vi "Get Time.vi"(8 "error in (no error)":errorcluster, 10 "Time Format (Absolute Time)":bool, 11 "VISA resource name":refnum<visa-resource-name>) -> (0 "error out":errorcluster, 1 "Current Time":string, 2 "Absolute Time":dbl format="%^#.8g", 3 "VISA resource name out":refnum<visa-resource-name>)   [LabVIEW 2020, in "Keithley 2450.lvlib"]
doc: "This gets the System Time in absolute or current time formats."
uses:
  Keithley 2450.lvlib
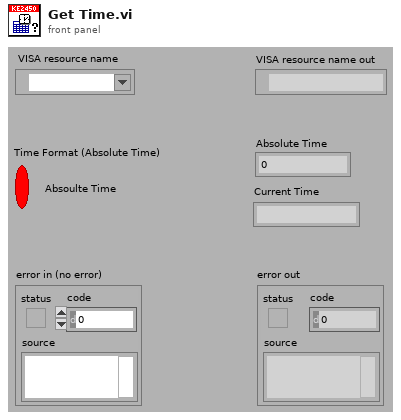
[diagram p1: front panel]
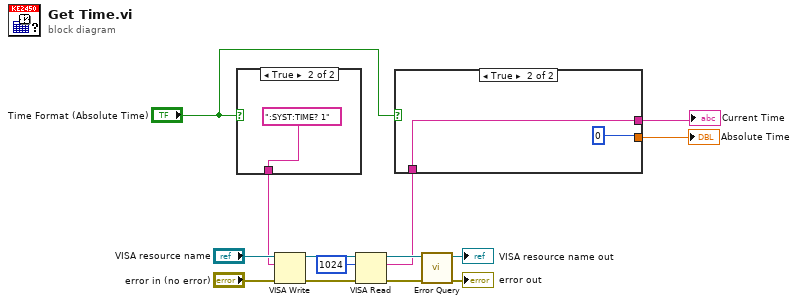
[diagram p0: block diagram]
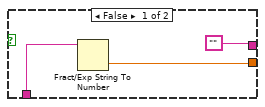
[diagram p2: hidden frame]
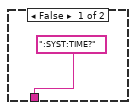
[diagram p3: hidden frame]
diagram:
  n1 = case shown="True" "Time Format (Absolute Time)" {
    tunnel: [":SYST:TIME?" ":SYST:TIME? 1"] -> w5
    frame False {
    }
    frame True {
    }
  }
  n2 = VISA Write(VISA resource name="VISA resource name", write buffer=w5, error in (no error)="error in (no error)") -> (VISA resource name out=w13:refnum<visa-resource-name>, error out=w14:errorcluster)  [unwired: 1 out]
  n3 = VISA Read(VISA resource name=w13, byte count=u32 1024, error in (no error)=w14) -> (VISA resource name out=w7:refnum<visa-resource-name>, read buffer=w4:string, error out=w6:errorcluster)  [unwired: 1 out]
  n4 = case shown="True" "Time Format (Absolute Time)" {
    tunnel: w4 -> [w19 w21]
    tunnel: ["" w21] -> w2
    tunnel: [w18 0] -> w1
    frame False {
      n5 = Fract/Exp String To Number(string=w19) -> (number=w18:dbl)  [unwired: 3 in, 1 out]
    }
    frame True {
    }
  }
  "Absolute Time" <- w1
  "Current Time" <- w2
  n6 = call "Error Query.vi"("error in (no error)"=w6, "VISA resource name"=w7) -> ("error out"=→"error out":errorcluster, "VISA resource name out"=→"VISA resource name out":refnum<visa-resource-name>)  [unwired: 8 out]
